vi "FTW-File-ResolveSymbolicPaths.vi"(0 "Unresolved Path":path, 11 "error in":errorcluster) -> (4 "Resolved Path":path, 15 "error out":errorcluster)   [LabVIEW 2013]
panel:
  # "Inputs"
  # "Outputs"
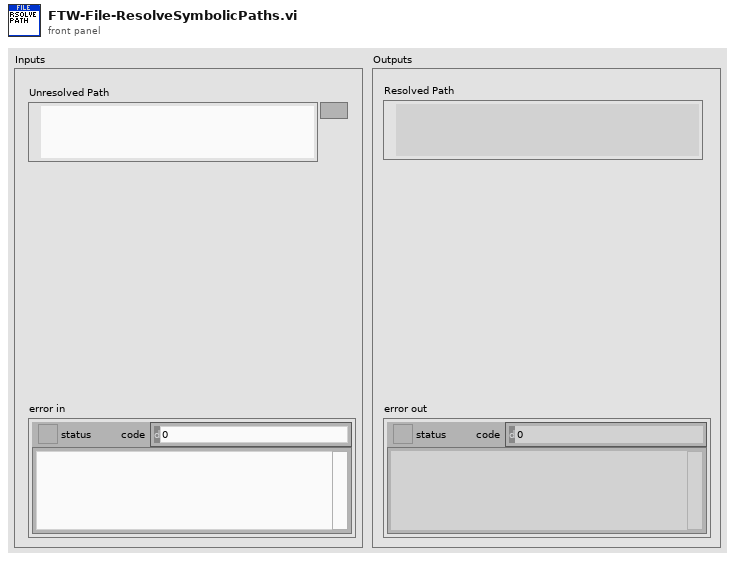
[diagram p1: front panel]
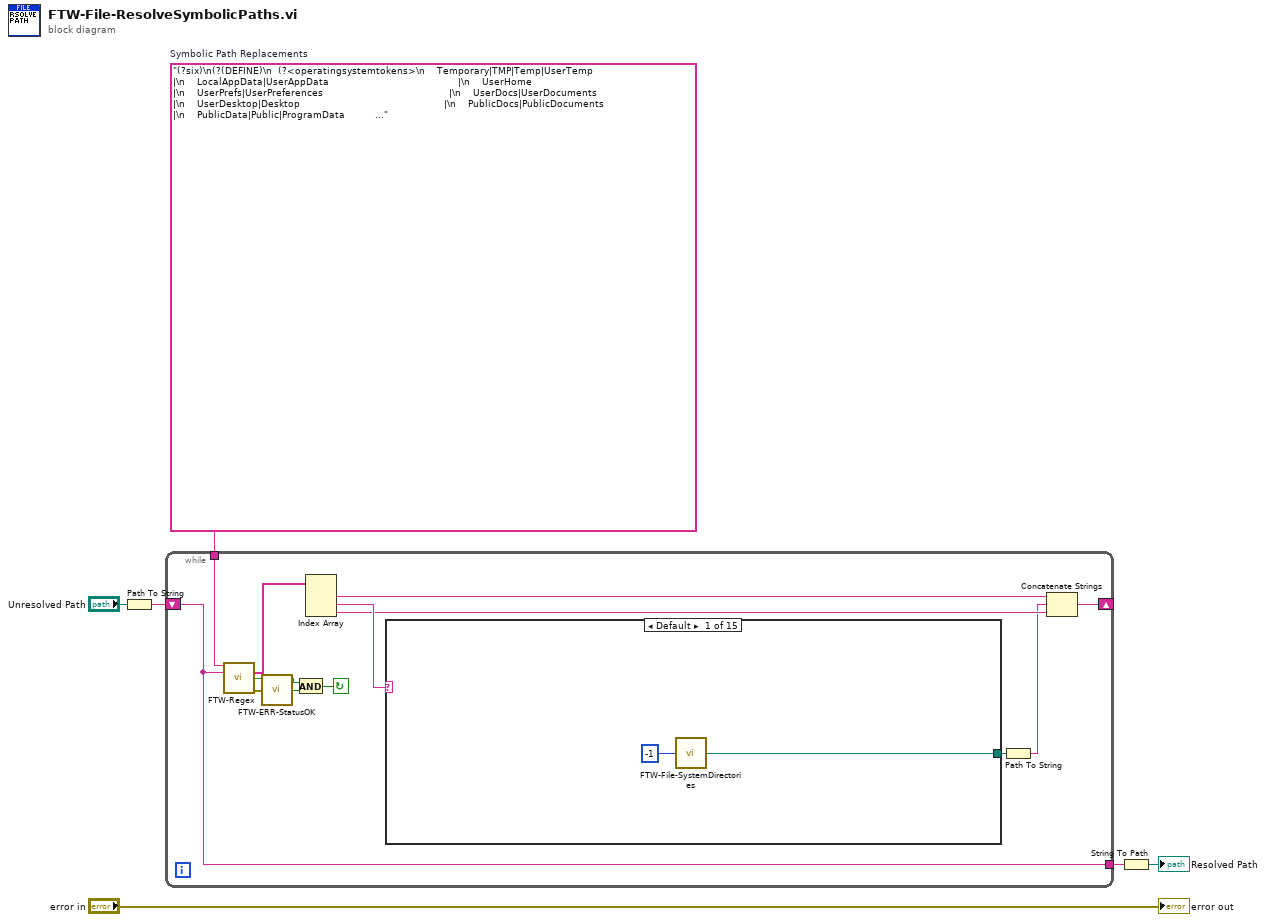
[diagram p0: block diagram]
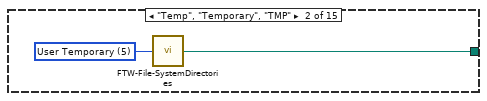
[diagram p2: hidden frame]
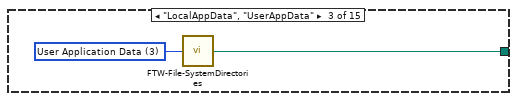
[diagram p3: hidden frame]
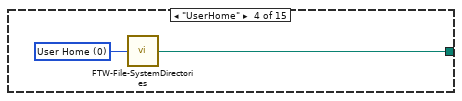
[diagram p4: hidden frame]
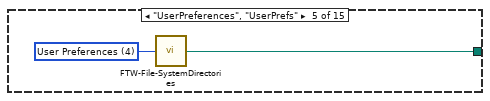
[diagram p5: hidden frame]
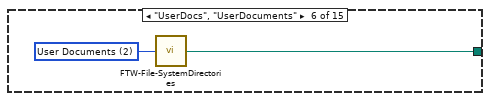
[diagram p6: hidden frame]
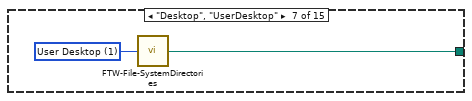
[diagram p7: hidden frame]
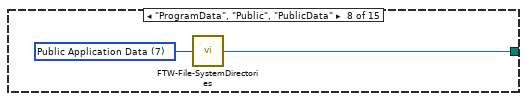
[diagram p8: hidden frame]
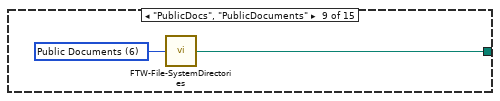
[diagram p9: hidden frame]
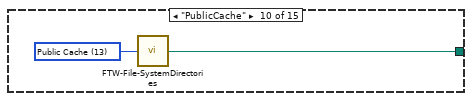
[diagram p10: hidden frame]
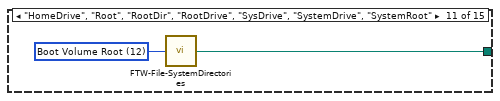
[diagram p11: hidden frame]
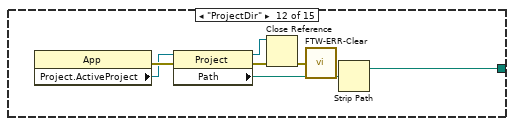
[diagram p12: hidden frame]
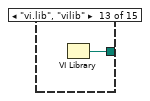
[diagram p13: hidden frame]
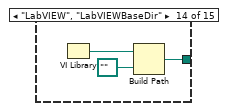
[diagram p14: hidden frame]
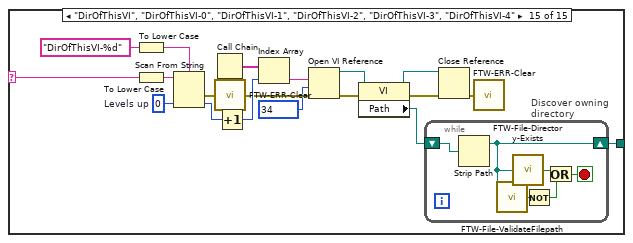
[diagram p15: hidden frame]
diagram:
  w3 = "(?six)\n(?(DEFINE)\n  (?<operatingsystemtokens>\n    Temporary|TMP|Temp|UserTemp                                        |\n    LocalAppData|UserAppData                                           |\n    UserHome                                                           |\n    UserPrefs|UserPreferences                                          |\n    UserDocs|UserDocuments                                             |\n    UserDesktop|Desktop                                                |\n    PublicDocs|PublicDocuments                                         |\n    PublicData|Public|ProgramData                                      |\n    RootDir|Root|SystemDrive|SysDrive|HomeDrive|RootDrive|SystemRoot\n  )\n  (?<labviewdirectorytokens>\n    ### LabVIEW-specific Tokens ###\n    ProjectDir                                                         |\n    resource                                                           |\n    vilib|vi\\.lib                                                      |\n    LabVIEWBaseDir|LabVIEW                                             |\n    DirOfThisVI(?:-[01234])?\n  )\n)\n\n### Allow OS tokens to be between [], %%, or <>\n### Allow LabVIEW tokens to be between [] or <>\n### Each symbolic path has an optional trailing colon (:)\n(\\A.*?)\n(?: \\[(  (?&operatingsystemtokens)  |  (?&labviewdirectorytokens)  )\\]:? |\n    \\<(  (?&operatingsystemtokens)  |  (?&labviewdirectorytokens)  )\\>:? |\n    \\%(  (?&operatingsystemtokens)                                 )\\%:? )\n(.*?\\z)"  # Symbolic Path Replacements
  n1 = Path To String(path="Unresolved Path") -> (string=w1:string)
  n2 = while {
    tunnel: w3 -> [w15]
    tunnel: [w12] -> w2
    shift-right: [w11] -> _
    shift-left: w1 -> [w12]
    stop <- w16 continue-if-true
    n3 = call "FTW-Regex.vi"("Regular Expression"=w15, "Input String"=w12) -> ("Submatches"=w14:string[], "Match Found?"=w18:bool, "error out"=w19:errorcluster)  [unwired: 9 in, 2 out]
    n4 = call "FTW-ERR-StatusOK.vi"("error to check"=w19) -> ("Status OK?"=w17:bool)
    n5 = And(x=w18, y=w17) -> (x .and. y?=w16:bool)
    n6 = Index Array(array=w14) -> (element #1=w10:string, element #2=w13:string, element #3=w9:string)  [unwired: 3 in]
    n7 = case shown="Default" w13 {
      selector: w13 -> [_ _ _ _ _ _ _ _ _ _ _ _ _ _ w71]
      tunnel: [w20 w23 w25 w27 w29 w31 w33 w34 w37 w38 w40 w42 w49 w51 w70] -> w7
      frame Default {
        n8 = call "FTW-File-SystemDirectories.vi"("System Directory"=-1) -> ("Directory"=w20:path)
      }
      frame "Temp", "Temporary", "TMP" {
        w22 = 5 items=["User Home"=0, "User Desktop"=1, "User Documents"=2, "User Application Data"=3, "User Preferences"=4, "User Temporary"=5, "Public Documents"=6, "Public Application Data"=7, "Public Preferences"=8, "Public Cache"=13, "System Core Libraries"=9, "System Installed Libraries"=10, "Application Files"=11, "Boot Volume Root"=12] ("System Directory")
        n9 = call "FTW-File-SystemDirectories.vi"("System Directory"=w22) -> ("Directory"=w23:path)
      }
      frame "LocalAppData", "UserAppData" {
        w24 = 3 items=["User Home"=0, "User Desktop"=1, "User Documents"=2, "User Application Data"=3, "User Preferences"=4, "User Temporary"=5, "Public Documents"=6, "Public Application Data"=7, "Public Preferences"=8, "Public Cache"=13, "System Core Libraries"=9, "System Installed Libraries"=10, "Application Files"=11, "Boot Volume Root"=12] ("System Directory")
        n10 = call "FTW-File-SystemDirectories.vi"("System Directory"=w24) -> ("Directory"=w25:path)
      }
      frame "UserHome" {
        w26 = 0 items=["User Home"=0, "User Desktop"=1, "User Documents"=2, "User Application Data"=3, "User Preferences"=4, "User Temporary"=5, "Public Documents"=6, "Public Application Data"=7, "Public Preferences"=8, "Public Cache"=13, "System Core Libraries"=9, "System Installed Libraries"=10, "Application Files"=11, "Boot Volume Root"=12] ("System Directory")
        n11 = call "FTW-File-SystemDirectories.vi"("System Directory"=w26) -> ("Directory"=w27:path)
      }
      frame "UserPreferences", "UserPrefs" {
        w28 = 4 items=["User Home"=0, "User Desktop"=1, "User Documents"=2, "User Application Data"=3, "User Preferences"=4, "User Temporary"=5, "Public Documents"=6, "Public Application Data"=7, "Public Preferences"=8, "Public Cache"=13, "System Core Libraries"=9, "System Installed Libraries"=10, "Application Files"=11, "Boot Volume Root"=12] ("System Directory")
        n12 = call "FTW-File-SystemDirectories.vi"("System Directory"=w28) -> ("Directory"=w29:path)
      }
      frame "UserDocs", "UserDocuments" {
        w30 = 2 items=["User Home"=0, "User Desktop"=1, "User Documents"=2, "User Application Data"=3, "User Preferences"=4, "User Temporary"=5, "Public Documents"=6, "Public Application Data"=7, "Public Preferences"=8, "Public Cache"=13, "System Core Libraries"=9, "System Installed Libraries"=10, "Application Files"=11, "Boot Volume Root"=12] ("System Directory")
        n13 = call "FTW-File-SystemDirectories.vi"("System Directory"=w30) -> ("Directory"=w31:path)
      }
      frame "Desktop", "UserDesktop" {
        w32 = 1 items=["User Home"=0, "User Desktop"=1, "User Documents"=2, "User Application Data"=3, "User Preferences"=4, "User Temporary"=5, "Public Documents"=6, "Public Application Data"=7, "Public Preferences"=8, "Public Cache"=13, "System Core Libraries"=9, "System Installed Libraries"=10, "Application Files"=11, "Boot Volume Root"=12] ("System Directory")
        n14 = call "FTW-File-SystemDirectories.vi"("System Directory"=w32) -> ("Directory"=w33:path)
      }
      frame "ProgramData", "Public", "PublicData" {
        w35 = 7 items=["User Home"=0, "User Desktop"=1, "User Documents"=2, "User Application Data"=3, "User Preferences"=4, "User Temporary"=5, "Public Documents"=6, "Public Application Data"=7, "Public Preferences"=8, "Public Cache"=13, "System Core Libraries"=9, "System Installed Libraries"=10, "Application Files"=11, "Boot Volume Root"=12] ("System Directory")
        n15 = call "FTW-File-SystemDirectories.vi"("System Directory"=w35) -> ("Directory"=w34:path)
      }
      frame "PublicDocs", "PublicDocuments" {
        w36 = 6 items=["User Home"=0, "User Desktop"=1, "User Documents"=2, "User Application Data"=3, "User Preferences"=4, "User Temporary"=5, "Public Documents"=6, "Public Application Data"=7, "Public Preferences"=8, "Public Cache"=13, "System Core Libraries"=9, "System Installed Libraries"=10, "Application Files"=11, "Boot Volume Root"=12] ("System Directory")
        n16 = call "FTW-File-SystemDirectories.vi"("System Directory"=w36) -> ("Directory"=w37:path)
      }
      frame "PublicCache" {
        w39 = 13 items=["User Home"=0, "User Desktop"=1, "User Documents"=2, "User Application Data"=3, "User Preferences"=4, "User Temporary"=5, "Public Documents"=6, "Public Application Data"=7, "Public Preferences"=8, "Public Cache"=13, "System Core Libraries"=9, "System Installed Libraries"=10, "Application Files"=11, "Boot Volume Root"=12] ("System Directory")
        n17 = call "FTW-File-SystemDirectories.vi"("System Directory"=w39) -> ("Directory"=w38:path)
      }
      frame "HomeDrive", "Root", "RootDir", "RootDrive", "SysDrive", "SystemDrive", "SystemRoot" {
        w41 = 12 items=["User Home"=0, "User Desktop"=1, "User Documents"=2, "User Application Data"=3, "User Preferences"=4, "User Temporary"=5, "Public Documents"=6, "Public Application Data"=7, "Public Preferences"=8, "Public Cache"=13, "System Core Libraries"=9, "System Installed Libraries"=10, "Application Files"=11, "Boot Volume Root"=12] ("System Directory")
        n18 = call "FTW-File-SystemDirectories.vi"("System Directory"=w41) -> ("Directory"=w40:path)
      }
      frame "ProjectDir" {
        n19 = property class="App"() -> (error out=w45:errorcluster, "Project.ActiveProject"=w44:refnum<vi>)  [unwired: 2 in, 1 out]
        n20 = property class="Project"(reference=w44, error in=w45) -> (reference out=w46:refnum<vi>, error out=w47:errorcluster, "Path"=w43:path)
        n21 = Close Reference(reference=w46, error in (no error)=w47) -> (error out=w48:errorcluster)
        n22 = call "FTW-ERR-Clear.vi"("error to snuff"=w48) -> ()  [unwired: 1 out]
        n23 = Strip Path(path=w43) -> (stripped path=w42:path)  [unwired: 1 out]
      }
      frame "vi.lib", "vilib" {
        n24 = VI Library() -> (path=w49:path)
      }
      frame "LabVIEW", "LabVIEWBaseDir" {
        n25 = VI Library() -> (path=w52:path)
        n26 = Build Path(base path=w52, name or relative path=path ".." ("appended path")) -> (appended path=w51:path)
      }
      frame "DirOfThisVI", "DirOfThisVI-0", "DirOfThisVI-1", "DirOfThisVI-2", "DirOfThisVI-3", "DirOfThisVI-4" {
        w63 = 0  # Levels up
        n27 = To Lower Case(string="DirOfThisVI-%d") -> (all lower case string=w54:string)
        n28 = To Lower Case(string=w71) -> (all lower case string=w57:string)
        n29 = Scan From String(format string=w54, input string=w57, default 1=w63) -> (error out=w60:errorcluster, output 1=w62:i32)  [unwired: 2 in, 2 out]
        n30 = Call Chain() -> (call chain=w67:string[])
        n31 = call "FTW-ERR-Clear.vi"("error to snuff"=w60) -> ("no error"=w59:errorcluster)
        n32 = Increment(x=w62) -> (x+1=w61:i32)
        n33 = Index Array(array=w67, index=w61) -> (element=w68:string)
        n34 = Open VI Reference(vi path=w68, options=34, error in (no error)=w59) -> (vi reference=w69:refnum<vi>, error out=w66:errorcluster)  [unwired: 3 in]
        n35 = property class="VI"(reference=w69, error in=w66) -> (reference out=w64:refnum<vi>, error out=w65:errorcluster, "Path"=w53:path)
        n36 = while "Discover owning directory" {
          shift-right: [w76] -> w70
          shift-left: w53 -> [w77]
          stop <- w74 stop-if-true
          n37 = Strip Path(path=w77) -> (stripped path=w76:path)  [unwired: 1 out]
          n38 = call "FTW-File-ValidateFilepath.vi"("Filepath"=w76) -> ("Valid?"=w73:bool)
          n39 = call "FTW-File-Directory-Exists.vi"("Directory"=w76) -> ("Exists?"=w75:bool)
          n40 = Not(x=w73) -> (.not. x?=w72:bool)
          n41 = Or(x=w75, y=w72) -> (x .or. y?=w74:bool)
        }
        n42 = Close Reference(reference=w64, error in (no error)=w65) -> (error out=w58:errorcluster)
        n43 = call "FTW-ERR-Clear.vi"("error to snuff"=w58) -> ()  [unwired: 1 out]
      }
    }
    n44 = Path To String(path=w7) -> (string=w8:string)
    n45 = Concatenate Strings(w10, w8, w9) -> (w11:string)
  }
  n46 = String To Path(string=w2) -> (path=→"Resolved Path":path)
  "error out" <- "error in"
